vi "Waveform Attribute, Set Current Time.vi"(6 "error in":errorcluster, 9 "waveform":waveform(dbl)) -> (0 "error out":errorcluster, 2 "Process Timestamp":dbl[unit] format="%.3f", 3 "waveform out":waveform(dbl), 4 "Date and Time":timestamp format="%<%.1X  %x>T")   [LabVIEW 2010]
doc: "The timestamp is the current time in seconds. LabVIEW calculates this timestamp using the number of seconds elapsed since 12:00 a.m., Friday, January 1, 1904, Universal Time [01-01-1904 00:00:00]."
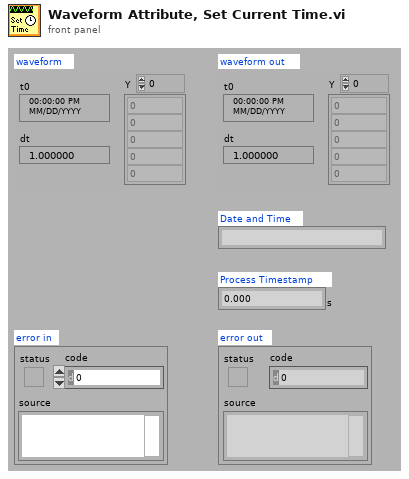
[diagram p1: front panel]
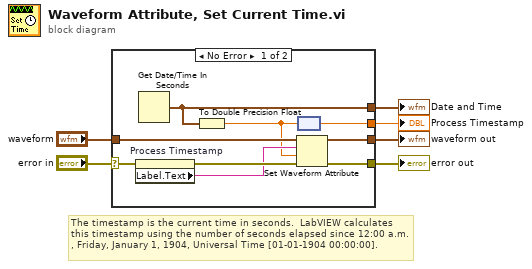
[diagram p0: block diagram]
diagram:
  # "The timestamp is the current time in seconds.  LabVIEW calculates this timestamp using the number of seconds elapsed since 12:00 a.m., Friday, January 1, 1904, Universal Time [01-01-1904 00:00:00]."
  n1 = case shown="No Error" "error in" {
    selector: "error in" -> [w11 w17]
    tunnel: [w15 w17] -> w6
    tunnel: "waveform" -> [w14 w16]
    tunnel: [w13 w16] -> w1
    tunnel: [w12 _] -> w4
    tunnel: [w8 _] -> w2
    frame No Error {
      n2 = property on="Process Timestamp" class="DigNum (strict)"(error in=w11) -> (error out=w10:errorcluster, "Label.Text"=w9:string)  [unwired: 1 in, 1 out]
      n3 = Get Date/Time In Seconds() -> (seconds since 1Jan1904=w12:timestamp)
      n4 = To Double Precision Float(number=w12) -> (double precision float=w7:dbl)
      n5 = Set Waveform Attribute(4:w10, 5:w7, 6:w9, 7:w14) -> (0:w15:errorcluster, 3:w13:waveform(dbl))  [unwired: 1 out]
      n6 = node(w7) -> (w8:dbl[unit])
    }
    frame Error {
    }
  }
  "error out" <- w6
  "waveform out" <- w1
  "Date and Time" <- w4
  "Process Timestamp" <- w2
